vi "SwissSPAD Live_Format SS2 U8 Data.vi"(8 "Error In":errorcluster, 9 "Y Resolution":i32=128, 10 "X Resolution":i32, 11 "Flattened Image":u8[](array[numeric])) -> (0 "Error Out":errorcluster, 3 "Image out":u8[][](array[numeric]))   [LabVIEW 2021]
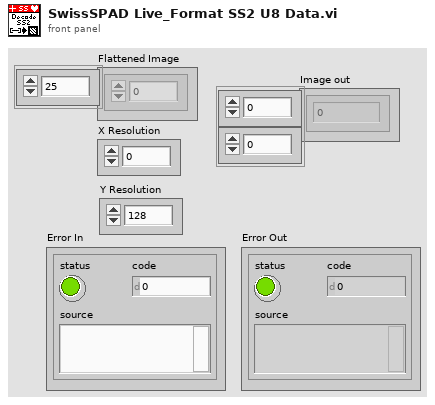
[diagram p1: front panel]
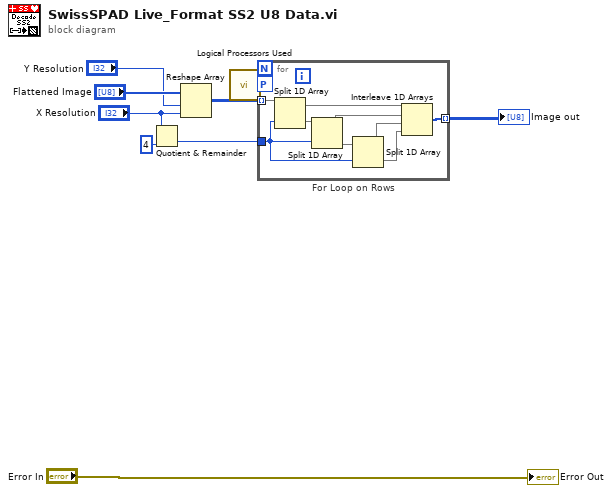
[diagram p0: block diagram]
diagram:
  n1 = Quotient & Remainder(x="X Resolution", y=4) -> (floor(x/y)=w3:i32)  [unwired: 1 out]
  n2 = Reshape Array("Flattened Image", "Y Resolution", "X Resolution") -> (w5:u8[][])
  n3 = call "Logical Processors Used.vi"() -> ("# Logical Processor Used"=w1:i32)  [unwired: 6 in]
  n4 = for "For Loop on Rows" {
    tunnel: w5 -> [w18] mode=indexing
    tunnel: w3 -> [w15]
    tunnel: [w10] -> w2 mode=indexing
    workers-P: w1 -> [_]
    n5 = Split 1D Array(array=w18, index=w15) -> (first subarray=w14:u8[], second subarray=w17:u8[])
    n6 = Split 1D Array(array=w17, index=w15) -> (first subarray=w13:u8[], second subarray=w16:u8[])
    n7 = Split 1D Array(array=w16, index=w15) -> (first subarray=w12:u8[], second subarray=w11:u8[])
    n8 = Interleave 1D Arrays(w14, w13, w12, w11) -> (w10:u8[])
  }
  "Image out" <- w2
  "Error Out" <- "Error In"
